vi "VisaWrite.vi"(0 "VISA资源名称":refnum<visa-resource-name>, 1 "command":string, 2 "Set Value":dbl format="%#_8g", 3 "错误输入（无错误）":errorcluster caption="错误输入", 4 "wP  w/oP":bool) -> (5 "错误输出":errorcluster)   [LabVIEW 2014]
panel:
  out "concatenated string":string
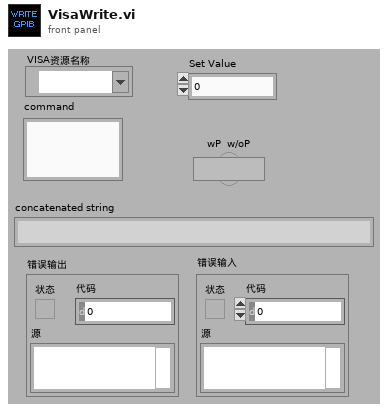
[diagram p1: front panel]
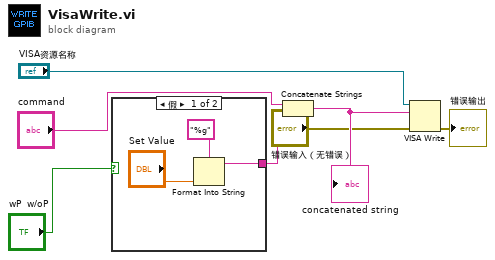
[diagram p0: block diagram]
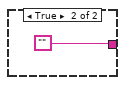
[diagram p2: hidden frame]
diagram:
  n1 = case shown="假" "wP  w/oP" {
    tunnel: [w9 ""] -> w7
    frame False {
      n2 = Format Into String(format string="%g" ("格式字符串"), "Set Value") -> (resulting string=w9:string)  [unwired: 2 in, 1 out]
    }
    frame True {
    }
  }
  n3 = Concatenate Strings("command", w7) -> (w6:string)
  "concatenated string" <- w6
  n4 = VISA Write(VISA resource name="VISA资源名称", write buffer=w6, error in (no error)="错误输入（无错误）") -> (error out=→"错误输出":errorcluster)  [unwired: 2 out]
